vi "FactoryExampleDEMO.vi"() -> ()   [LabVIEW 2013]
uses:
  USB-9215/USB-9215.lvclass
  USB-9234/USB-9234.lvclass
  DAQSuper/DAQSuper.lvclass
panel:
  out "Waveform Graph":waveform(dbl)(graph)
  out "MaxSampleClock":dbl
  out "ChannelCount":dbl
  out "DeviceName":string
  in  "DeviceSelect":enum16{"USB-9215", "USB-9234"}(ring)
  # "工廠模式簡例\n1. 定義抽象class\"DAQSuper\"\n     具有GetDeviceInfo與GetData行為方法，但不實作內部CODE\n\n2. 定義具體clsss\"USB-9215\"與\"USB-9234\"繼承自抽象class\"DAQSuper\"\n    並Override實作\"USB-9215\"與\"USB-9234\"\n    兩者各自的 GetDeviceInfo與GetData行為方法的CODE\n\n3. 在執行階段選擇載入\"USB-9215\"或\"USB-9234\"\n    並執行 GetDeviceInfo與GetData行為方法\n\n4. 若欲增加其它卡種，只要重做步驟2即可，不影響即有卡種class的程式"
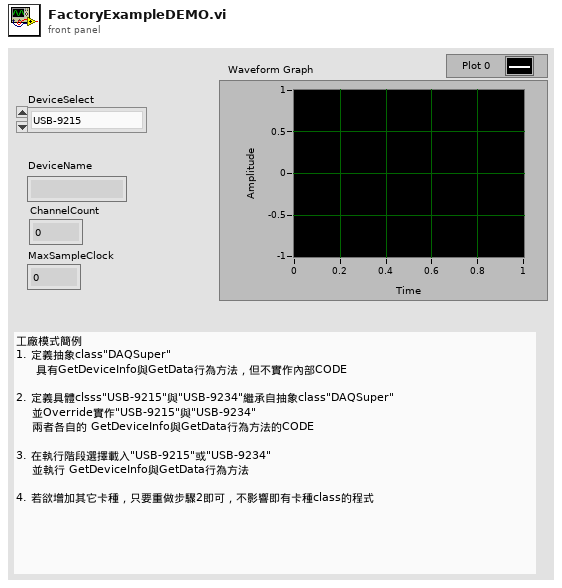
[diagram p1: front panel]
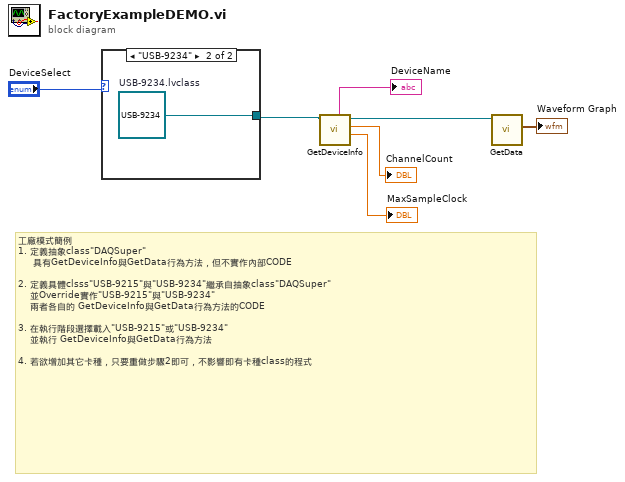
[diagram p0: block diagram]
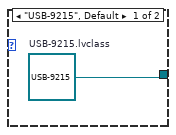
[diagram p2: hidden frame]
diagram:
  # "工廠模式簡例\n1. 定義抽象class\"DAQSuper\"\n     具有GetDeviceInfo與GetData行為方法，但不實作內部CODE\n\n2. 定義具體clsss\"USB-9215\"與\"USB-9234\"繼承自抽象class\"DAQSuper\"\n    並Override實作\"USB-9215\"與\"USB-9234\"\n    兩者各自的 GetDeviceInfo與GetData行為方法的CODE\n\n3. 在執行階段選擇載入\"USB-9215\"或\"USB-9234\"\n    並執行 GetDeviceInfo與GetData行為方法\n\n4. 若欲增加其它卡種，只要重做步驟2即可，不影響即有卡種class的程式"
  n1 = case shown="\"USB-9234\"" "DeviceSelect" {
    tunnel: [w8 w9] -> w6
    frame "USB-9215", Default {
      w8 = refnum<class "USB-9215.lvclass"> refnum  # USB-9215.lvclass
    }
    frame "USB-9234" {
      w9 = refnum<class "USB-9234.lvclass"> refnum  # USB-9234.lvclass
    }
  }
  n2 = call-dynamic "GetDeviceInfo.vi"("DAQSuper in"=w6) -> ("MaxSampleClock"=→"MaxSampleClock":dbl, "ChannelCount"=→"ChannelCount":dbl, "DAQSuper out"=w2:refnum<class "DAQSuper.lvclass">, "DeviceName"=→"DeviceName":string)  [unwired: 6 in, 1 out]
  n3 = call-dynamic "GetData.vi"("DAQSuper in"=w2) -> ("Waveform"=→"Waveform Graph":waveform(dbl))  [unwired: 8 in, 2 out]
